vi "parseXMLstring.vi"(8 "error in (no error)":errorcluster, 10 "Node Value":string, 11 "Experiment.lvclass (in)":refnum<class "Experiment.lvclass">) -> (0 "error out":errorcluster, 3 "Experiment.lvclass":refnum<class "Experiment.lvclass">)   [LabVIEW 2013, in "Experiment.lvclass"]
uses:
  Experiment/Experiment.lvclass
  Experiment/states.ctl
  Experiment/Experiment.lvclass/Experiment.ctl
  DDS/DDS.lvclass
  HSDIO/HSDIO.lvclass
  ExperimentVariables/ExperimentVariables.lvclass
  Camera/Hamamatsu_C9100-13/Hamamatsu_C9100-13.lvclass
  Analog_output/Analog_Output.lvclass
  PI_piezo/PI_Piezo.lvclass
  Experiment/Globals.vi
  <vilib>/xml/Close Reference(Node).vi
  <vilib>/xml/NI_XML.lvlib
  <resource>/objmgr/DOMUserDefRef.rc
  GPIB/GPIB.lvclass
  TCP_IP.lvclass
panel:
  out "Parse Errors":string
  out "Display of element names":string[](array[string])
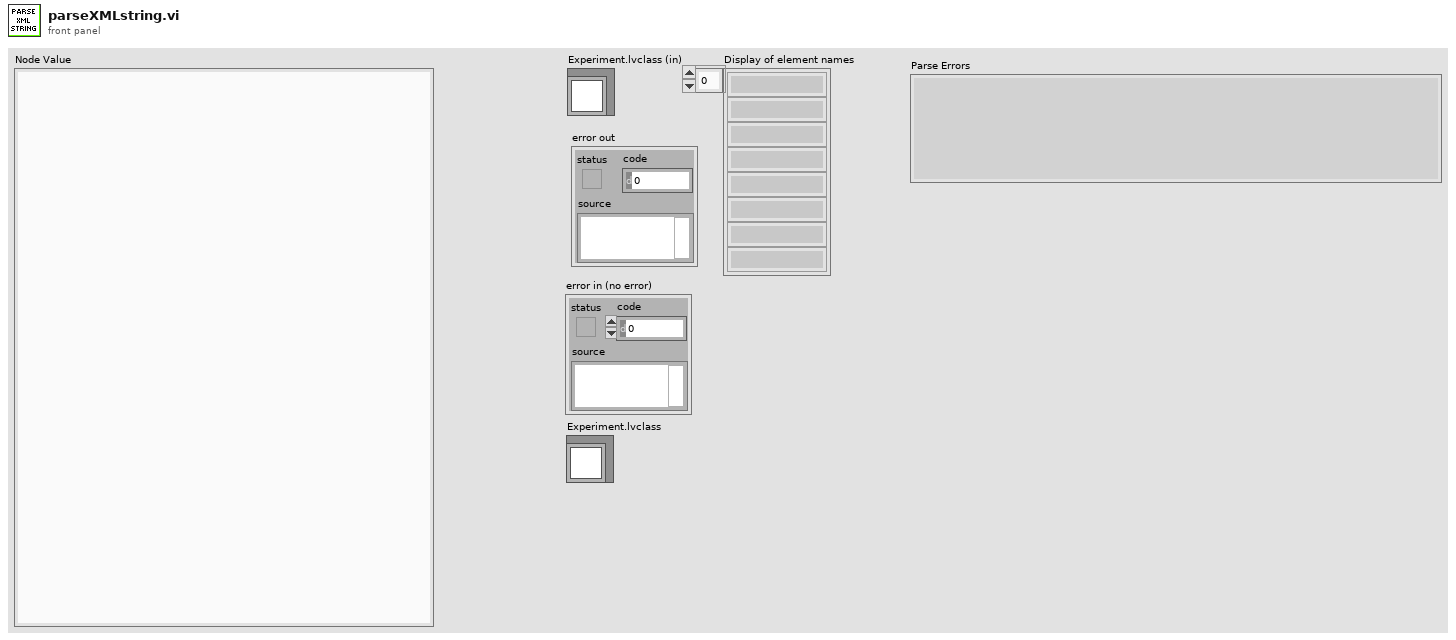
[diagram p1: front panel]
types:
  T1 = typedef "states.ctl" = enum16{"run", "pause", "shutdown gracefully", "halt immediately", "waiting for connection", "waiting for command"}
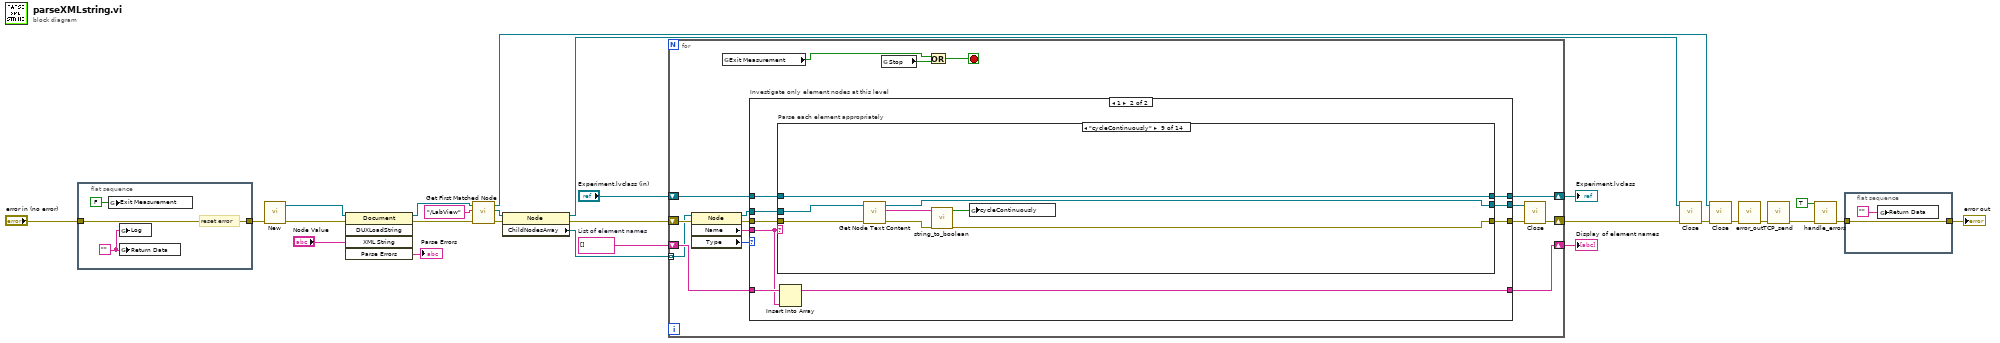
[diagram p0: block diagram]
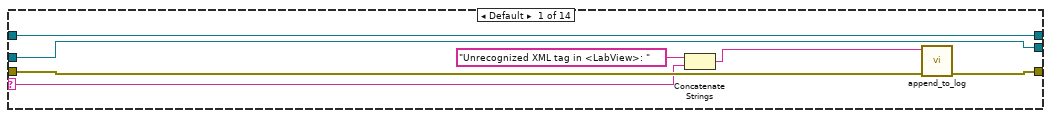
[diagram p3: hidden frame]
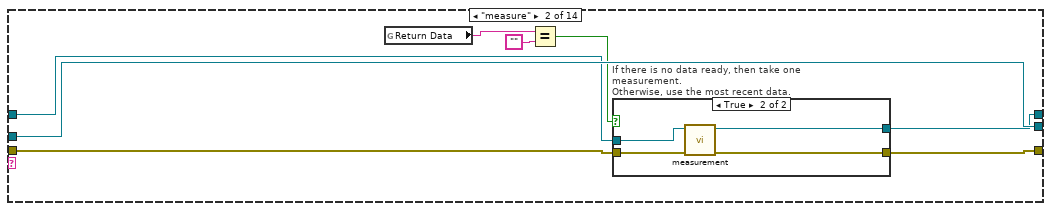
[diagram p4: hidden frame]
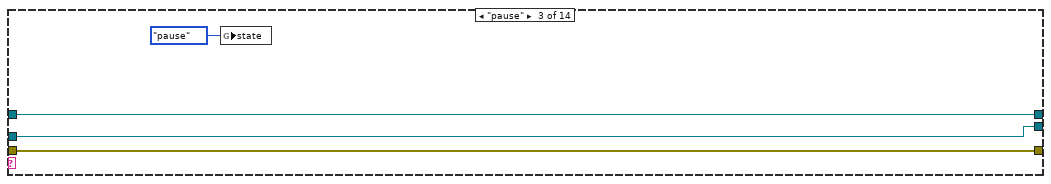
[diagram p6: hidden frame]
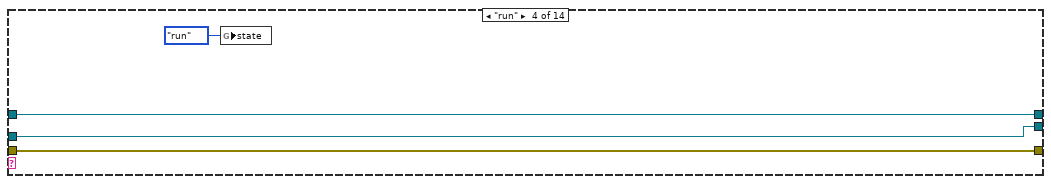
[diagram p7: hidden frame]
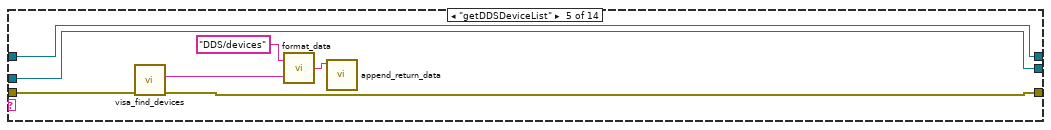
[diagram p8: hidden frame]
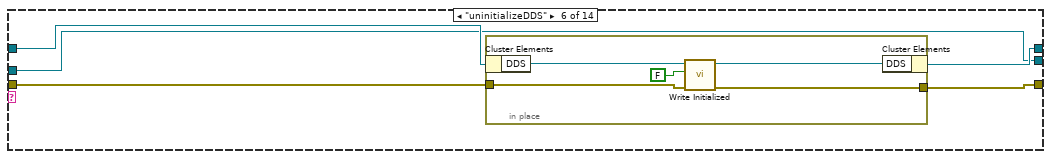
[diagram p9: hidden frame]
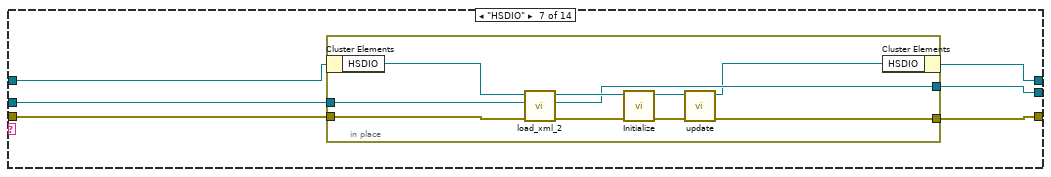
[diagram p10: hidden frame]
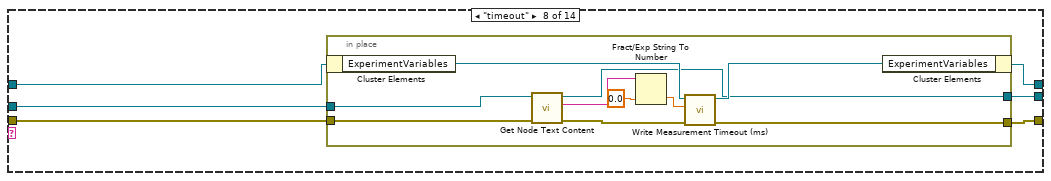
[diagram p11: hidden frame]
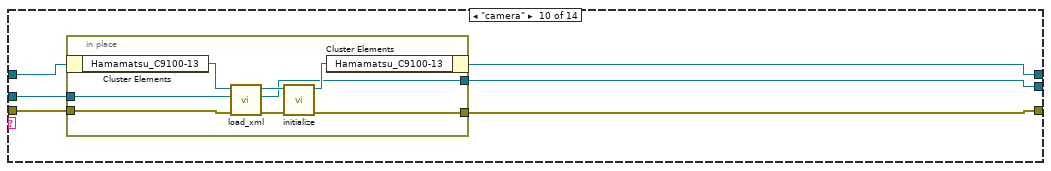
[diagram p12: hidden frame]
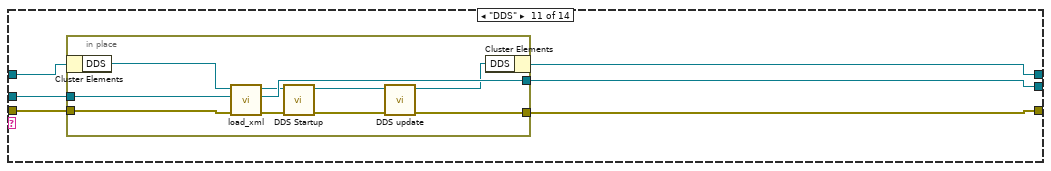
[diagram p13: hidden frame]
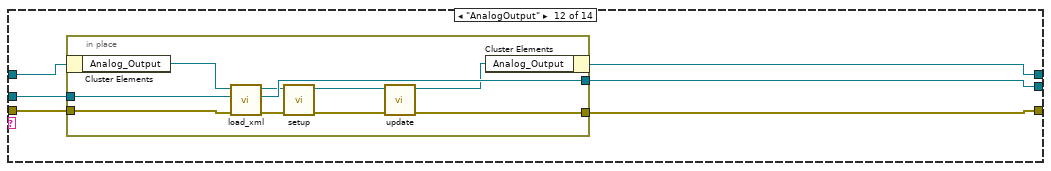
[diagram p14: hidden frame]
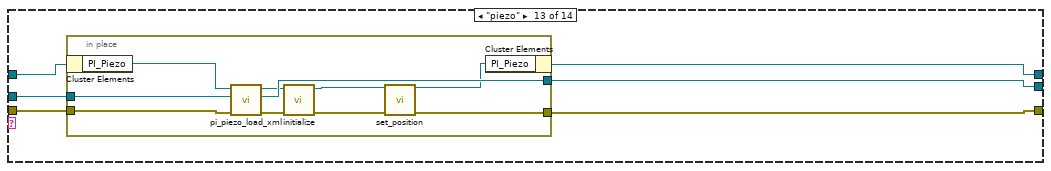
[diagram p15: hidden frame]
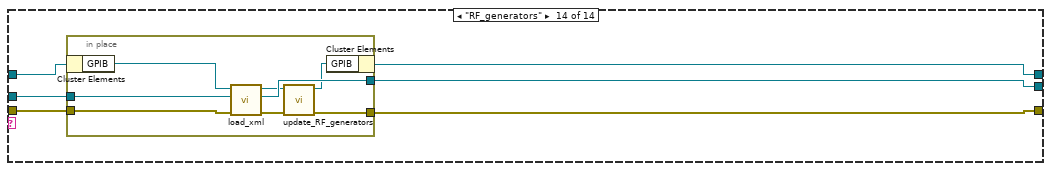
[diagram p16: hidden frame]
diagram:
  w19 = string[] []  # List of element names
  n1 = flat-sequence {
    tunnel: "error in (no error)" -> [w30]
    tunnel: [w30] -> w7
    frame #0 {
      w28 = ""
      # "reset error"
      n2 = global write "Globals.vi" "Exit Measurement"(FALSE ("Exit Measurement")) -> ()
      n3 = global write "Globals.vi" "Log"(w28) -> ()
      n4 = global write "Globals.vi" "Return Data"(w28) -> ()
    }
  }
  n5 = call <vilib>:"New.vi"("error in (no error)"=w7) -> ("error out"=w12:errorcluster, "DOM document out"=w20:refnum<k20>)  [unwired: 7 in]
  n6 = invoke class="Document" method="DUXLoadString"(reference=w20, error in=w12, "XML String"="Node Value") -> (reference out=w23:refnum<k20>, error out=w11:errorcluster, "Parse Errors"=→"Parse Errors":string)  [unwired: 2 in, 2 out]
  n7 = call <vilib>:"Get First Matched Node.vi"("error in (no error)"=w11, "XPath expression"="/LabView", "node in"=w23) -> ("error out"=w17:errorcluster, "node result"=w13:refnum<k20>, "node out"=w18:refnum<k20>)  [unwired: 6 in]
  n8 = property class="Node"(reference=w13, error in=w17) -> (reference out=w21:refnum<k20>, error out=w15:errorcluster, "ChildNodesArray"=w27:refnum<k20>[])
  n9 = for {
    tunnel: w27 -> [w40] mode=indexing
    shift-right: [w43] -> w26
    shift-left: w19 -> [w44]
    shift-right: [w42] -> w16
    shift-left: w15 -> [w41]
    shift-right: [w34] -> w9
    shift-left: "Experiment.lvclass (in)" -> [w35]
    stop <- w31 stop-if-true
    n10 = property class="Node"(reference=w40, error in=w41) -> (reference out=w37:refnum<k20>, error out=w39:errorcluster, "Name"=w45:string, "Type"=w46:i32)
    n11 = global read "Globals.vi" "Exit Measurement"() -> (w33:bool)
    n12 = case "Investigate only element nodes at this level" shown="1" w46 {
      tunnel: w45 -> [_ w57]
      tunnel: w44 -> [w50 w59]
      tunnel: [w50 w58] -> w43
      tunnel: w37 -> [w48 w56]
      tunnel: w39 -> [w49 w55]
      tunnel: [w49 w54] -> w38
      tunnel: [w48 w53] -> w36
      tunnel: w35 -> [w47 w52]
      tunnel: [w47 w51] -> w34
      frame Default {
      }
      frame 1 {
        n13 = case "Parse each element appropriately" shown="\"cycleContinuously\"" w57 {
          selector: w57 -> [w63 _ _ _ _ _ _ _ _ _ _ _ _ _]
          tunnel: w56 -> [w61 w74 w81 w85 w92 w96 w107 w123 w145 w147 w161 w177 w193 w209]
          tunnel: w55 -> [w66 w70 w82 w86 w91 w98 w109 w125 w141 w148 w162 w178 w194 w210]
          tunnel: [w65 w69 w82 w86 w90 w97 w108 w124 w140 w149 w163 w179 w195 w211] -> w54
          tunnel: [w61 w74 w81 w85 w92 w96 w106 w122 w142 w146 w160 w176 w192 w208] -> w53
          tunnel: w52 -> [w60 w68 w83 w87 w93 w100 w111 w127 w138 w151 w165 w181 w197 w213]
          tunnel: [w60 w67 w83 w87 w93 w99 w110 w126 w138 w150 w164 w180 w196 w212] -> w51
          frame Default {
            n14 = Concatenate Strings("Unrecognized XML tag in <LabView>: " ("string"), w63) -> (w62:string)
            n15 = call "append_to_log.vi"("error in"=w66, "string"=w62) -> ("error out"=w65:errorcluster)  [unwired: 9 in]
          }
          frame "measure" {
            n16 = global read "Globals.vi" "Return Data"() -> (w73:string)
            n17 = Equal?(x=w73, y="") -> (x = y?=w71:bool)
            n18 = case "If there is no data ready, then take one measurement.\nOtherwise, use the most recent data." shown="True" w71 {
              tunnel: w70 -> [w76 w80]
              tunnel: [w76 w79] -> w69
              tunnel: w68 -> [w75 w78]
              tunnel: [w75 w77] -> w67
              frame False {
              }
              frame True {
                n19 = call "measurement.vi"("error in (no error)"=w80, "Experiment.lvclass"=w78) -> ("error out"=w79:errorcluster, "Experiment out"=w77:refnum<class "Experiment.lvclass">)  [unwired: 6 in]
              }
            }
          }
          frame "pause" {
            n20 = global write "Globals.vi" "state"(states."pause" ("state")) -> ()
          }
          frame "run" {
            n21 = global write "Globals.vi" "state"(states."run" ("state")) -> ()
          }
          frame "getDDSDeviceList" {
            n22 = call "visa_find_devices.vi"("error in (no error)"=w91) -> ("error out"=w90:errorcluster, "devices found string"=w89:string)  [unwired: 8 in, 1 out]
            n23 = call "format_data.vi"("data"=w89, "name"="DDS/devices") -> ("concatenated string"=w94:string)
            n24 = call "append_return_data.vi"("Return Data"=w94) -> ()  [unwired: 11 in]
          }
          frame "uninitializeDDS" {
            n25 = in-place {
              in-place-border: w98 -> [w102]
              in-place-border: [w101] -> w97
              n26 = in-place-cluster #1(w100) -> ("DDS"=w105:refnum<class "DDS.lvclass">)
              n27 = call-dynamic "Write Initialized.vi"("error in (no error)"=w102, "Initialized"=FALSE, "DDS in"=w105) -> ("error out"=w101:errorcluster, "DDS out"=w104:refnum<class "DDS.lvclass">)  [unwired: 7 in]
              n28 = in-place-cluster #1("DDS"=w104) -> (w99:refnum<class "Experiment.lvclass">)
            }
          }
          frame "HSDIO" {
            n29 = in-place {
              in-place-border: w109 -> [w120]
              in-place-border: [w113] -> w108
              in-place-border: w107 -> [w121]
              in-place-border: [w116] -> w106
              n30 = in-place-cluster #2(w111) -> ("HSDIO"=w119:refnum<class "HSDIO.lvclass">)
              n31 = call "load_xml_2.vi"("error in"=w120, "child node in"=w121, "HSDIO (in)"=w119) -> ("error out"=w117:errorcluster, "child node out"=w116:refnum<k20>, "HSDIO"=w118:refnum<class "HSDIO.lvclass">)  [unwired: 6 in]
              n32 = call "Initialize.vi"("error in (no error)"=w117, "HSDIO in"=w118) -> ("error out"=w114:errorcluster, "HSDIO out"=w115:refnum<class "HSDIO.lvclass">)  [unwired: 8 in]
              n33 = call-dynamic "update.vi"("error in (no error)"=w114, "HSDIO in"=w115) -> ("error out"=w113:errorcluster, "HSDIO out"=w112:refnum<class "HSDIO.lvclass">)  [unwired: 8 in]
              n34 = in-place-cluster #2("HSDIO"=w112) -> (w110:refnum<class "Experiment.lvclass">)
            }
          }
          frame "timeout" {
            n35 = in-place {
              in-place-border: w125 -> [w133]
              in-place-border: [w135] -> w124
              in-place-border: w123 -> [w134]
              in-place-border: [w131] -> w122
              n36 = in-place-cluster #3(w127) -> ("ExperimentVariables"=w137:refnum<class "ExperimentVariables.lvclass">)
              n37 = call <vilib>:"Get Node Text Content.vi"("error in (no error)"=w133, "node in"=w134) -> ("error out"=w132:errorcluster, "node text"=w129:string, "node out"=w131:refnum<k20>)  [unwired: 7 in]
              n38 = Fract/Exp String To Number(string=w129, default (0 dbl)=0.0 ("default (0 I32)")) -> (number=w128:dbl)  [unwired: 2 in, 1 out]
              n39 = call-dynamic "Write Measurement Timeout (ms).vi"("error in (no error)"=w132, "Measurement Timeout (ms)"=w128, "ExperimentVariables in"=w137) -> ("error out"=w135:errorcluster, "ExperimentVariables out"=w136:refnum<class "ExperimentVariables.lvclass">)  [unwired: 7 in]
              n40 = in-place-cluster #3("ExperimentVariables"=w136) -> (w126:refnum<class "Experiment.lvclass">)
            }
          }
          frame "cycleContinuously" {
            n41 = call <vilib>:"Get Node Text Content.vi"("error in (no error)"=w141, "node in"=w145) -> ("error out"=w144:errorcluster, "node text"=w143:string, "node out"=w142:refnum<k20>)  [unwired: 7 in]
            n42 = call "string_to_boolean.vi"("error in"=w144, "string"=w143) -> ("error out"=w140:errorcluster, "boolean"=w139:bool)  [unwired: 8 in]
            n43 = global write "Globals.vi" "cycleContinuously"(w139) -> ()
          }
          frame "camera" {
            n44 = in-place {
              in-place-border: [w155] -> w149
              in-place-border: w148 -> [w154]
              in-place-border: w147 -> [w153]
              in-place-border: [w152] -> w146
              n45 = in-place-cluster #4(w151) -> ("Hamamatsu_C9100-13"=w158:refnum<class "Hamamatsu_C9100-13.lvclass">)
              n46 = call "load_xml.vi"("error in"=w154, "child node in"=w153, "Hamamatsu_C9100-13.lvclass (in)"=w158) -> ("error out"=w156:errorcluster, "child node out"=w152:refnum<k20>, "Hamamatsu_C9100-13.lvclass"=w157:refnum<class "Hamamatsu_C9100-13.lvclass">)  [unwired: 6 in]
              n47 = call-dynamic "initialize.vi"("error in (no error)"=w156, "Hamamatsu_C9100-13 in"=w157) -> ("error out"=w155:errorcluster, "Hamamatsu_C9100-13 out"=w159:refnum<class "Hamamatsu_C9100-13.lvclass">)  [unwired: 8 in]
              n48 = in-place-cluster #4("Hamamatsu_C9100-13"=w159) -> (w150:refnum<class "Experiment.lvclass">)
            }
          }
          frame "DDS" {
            n49 = in-place {
              in-place-border: [w170] -> w163
              in-place-border: w162 -> [w173]
              in-place-border: w161 -> [w174]
              in-place-border: [w172] -> w160
              n50 = in-place-cluster #5(w165) -> ("DDS"=w175:refnum<class "DDS.lvclass">)
              n51 = call "load_xml.vi"("error in"=w173, "child node in"=w174, "DDS.lvclass (in)"=w175) -> ("error out"=w168:errorcluster, "child node out"=w172:refnum<k20>, "DDS.lvclass"=w169:refnum<class "DDS.lvclass">)  [unwired: 6 in]
              n52 = call "DDS Startup.vi"("error in (no error)"=w168, "DDS.lvclass (in)"=w169) -> ("error out"=w167:errorcluster, "DDS.lvclass"=w166:refnum<class "DDS.lvclass">)  [unwired: 8 in]
              n53 = call "DDS update.vi"("error in (no error)"=w167, "DDS.lvclass (in)"=w166) -> ("error out"=w170:errorcluster, "DDS.lvclass"=w171:refnum<class "DDS.lvclass">)  [unwired: 8 in]
              n54 = in-place-cluster #5("DDS"=w171) -> (w164:refnum<class "Experiment.lvclass">)
            }
          }
          frame "AnalogOutput" {
            n55 = in-place {
              in-place-border: [w185] -> w179
              in-place-border: w178 -> [w189]
              in-place-border: w177 -> [w190]
              in-place-border: [w188] -> w176
              n56 = in-place-cluster #6(w181) -> ("Analog_Output"=w191:refnum<class "Analog_Output.lvclass">)
              n57 = call "load_xml.vi"("error in"=w189, "child node in"=w190, "Analog_Output.lvclass (in)"=w191) -> ("error out"=w187:errorcluster, "child node out"=w188:refnum<k20>, "Analog_Output.lvclass"=w184:refnum<class "Analog_Output.lvclass">)  [unwired: 6 in]
              n58 = call "setup.vi"("error in (no error)"=w187, "Analog_Output in"=w184) -> ("error out"=w186:errorcluster, "Analog_Output out"=w183:refnum<class "Analog_Output.lvclass">)  [unwired: 8 in]
              n59 = call-dynamic "update.vi"("error in (no error)"=w186, "Analog_Output in"=w183) -> ("error out"=w185:errorcluster, "Analog_Output out"=w182:refnum<class "Analog_Output.lvclass">)  [unwired: 8 in]
              n60 = in-place-cluster #6("Analog_Output"=w182) -> (w180:refnum<class "Experiment.lvclass">)
            }
          }
          frame "piezo" {
            n61 = in-place {
              in-place-border: [w199] -> w195
              in-place-border: w194 -> [w205]
              in-place-border: w193 -> [w206]
              in-place-border: [w204] -> w192
              n62 = in-place-cluster #7(w197) -> ("PI_Piezo"=w207:refnum<class "PI_Piezo.lvclass">)
              n63 = call "pi_piezo_load_xml.vi"("error in"=w205, "child node in"=w206, "PI_Piezo (in)"=w207) -> ("error out"=w202:errorcluster, "child node out"=w204:refnum<k20>, "PI_Piezo"=w203:refnum<class "PI_Piezo.lvclass">)  [unwired: 6 in]
              n64 = call-dynamic "initialize.vi"("error in (no error)"=w202, "PI_Piezo in"=w203) -> ("error out"=w198:errorcluster, "PI_Piezo out"=w201:refnum<class "PI_Piezo.lvclass">)  [unwired: 8 in]
              n65 = call "set_position.vi"("PI_Piezo (in)"=w201, "error in"=w198) -> ("PI_Piezo"=w200:refnum<class "PI_Piezo.lvclass">, "error out"=w199:errorcluster)  [unwired: 12 in]
              n66 = in-place-cluster #7("PI_Piezo"=w200) -> (w196:refnum<class "Experiment.lvclass">)
            }
          }
          frame "RF_generators" {
            n67 = in-place {
              in-place-border: [w218] -> w211
              in-place-border: w210 -> [w220]
              in-place-border: w209 -> [w219]
              in-place-border: [w217] -> w208
              n68 = in-place-cluster #8(w213) -> ("GPIB"=w221:refnum<class "GPIB.lvclass">)
              n69 = call "load_xml.vi"("error in"=w220, "child node in"=w219, "GPIB (in)"=w221) -> ("error out"=w216:errorcluster, "child node out"=w217:refnum<k20>, "GPIB"=w215:refnum<class "GPIB.lvclass">)  [unwired: 6 in]
              n70 = call "update_RF_generators.vi"("error in"=w216, "GPIB (in)"=w215) -> ("error out"=w218:errorcluster, "GPIB"=w214:refnum<class "GPIB.lvclass">)  [unwired: 8 in]
              n71 = in-place-cluster #8("GPIB"=w214) -> (w212:refnum<class "Experiment.lvclass">)
            }
          }
        }
        n72 = Insert Into Array(array=w59, new element=w57) -> (w58:string[])  [unwired: 1 in]
      }
    }
    n73 = global read "Globals.vi" "Stop"() -> (w32:bool)
    n74 = Or(x=w33, y=w32) -> (x .or. y?=w31:bool)
    n75 = call-poly <vilib>:"Close.vi"("error in (no error)"=w38, "node"=w36) -> ("error out"=w42:errorcluster)  [unwired: 7 in]
  }
  "Display of element names" <- w26
  "Experiment.lvclass" <- w9
  n76 = call-poly <vilib>:"Close.vi"("error in (no error)"=w16, "node"=w21) -> ("error out"=w14:errorcluster)  [unwired: 7 in]
  n77 = call-poly <vilib>:"Close.vi"("error in (no error)"=w14, "node"=w18) -> ("error out"=w5:errorcluster)  [unwired: 7 in]
  n78 = call "error_out.vi"("error in (no error)"=w5) -> ("error out"=w6:errorcluster)  [unwired: 10 in]
  n79 = call "TCP_send.vi"("error in (no error)"=w6) -> ("error out"=w4:errorcluster)  [unwired: 10 in]
  n80 = call "handle_errors.vi"("Exit Operation"=TRUE ("Exit Measurement"), "error in (no error)"=w4) -> ("error out"=w1:errorcluster)  [unwired: 13 in]
  n81 = flat-sequence {
    tunnel: [w222] -> w2
    tunnel: w1 -> [w222]
    frame #0 {
      n82 = global write "Globals.vi" "Return Data"("") -> ()
    }
  }
  "error out" <- w2
